vi "test-Vision-Utils-ALL-TESTS.vi"(8 "error in (no error)":errorcluster) -> (0 "error out":errorcluster, 3 "All Passed":bool)   [LabVIEW 2019]
panel:
  out "Test 1":bool
  out "Test 1":bool
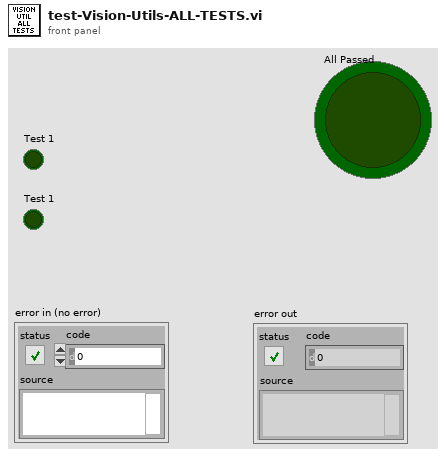
[diagram p1: front panel]
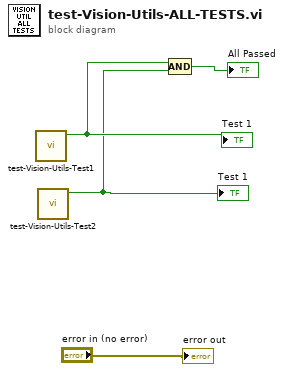
[diagram p0: block diagram]
diagram:
  n1 = call "test-Vision-Utils-Test1.vi"() -> ("All Passed"=w2:bool)  [unwired: 11 in]
  "Test 1" <- w2
  n2 = call "test-Vision-Utils-Test2.vi"() -> ("All Passed"=w1:bool)  [unwired: 11 in]
  "Test 1" <- w1
  n3 = Compound Arithmetic op=AND(w2, w1) -> (→"All Passed":bool)
  "error out" <- "error in (no error)"
